vi "add_log_entry.vi"(5 "new entry":string, 6 "error in (no error)":errorcluster, 8 "log identifiers":string(combo), 9 "StatusLog in":refnum<class "StatusLog.lvclass">) -> (0 "error out":errorcluster, 3 "StatusLog out":refnum<class "StatusLog.lvclass">)   [LabVIEW 2017, in "StatusLog.lvclass"]
doc: "adds a new log entry to the logfile. The path to the logfile is internally determined"
uses:
  StatusLog.lvclass
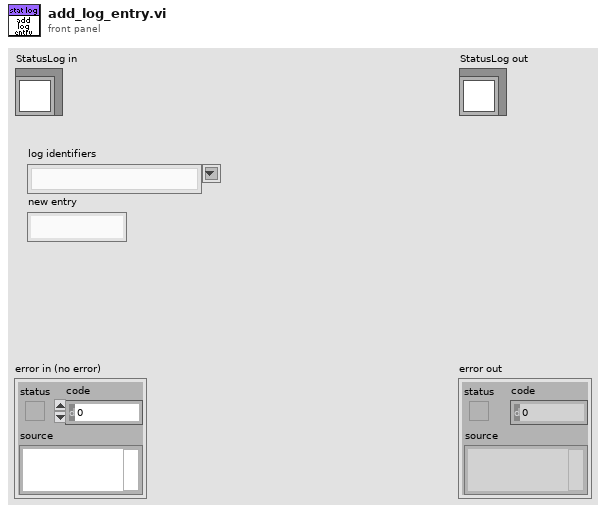
[diagram p1: front panel]
types:
  T1 = enum16{"open", "replace", "create", "open or create", "replace or create", "replace or create with confirmation"}
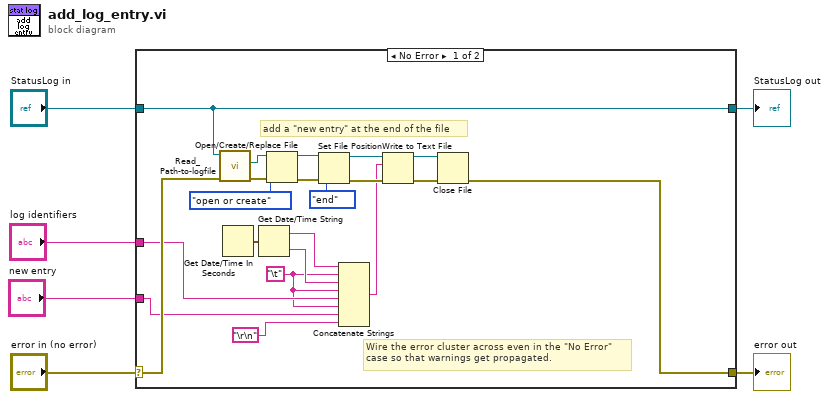
[diagram p0: block diagram]
diagram:
  n1 = case shown="No Error" "error in (no error)" {
    selector: "error in (no error)" -> [w17 w29]
    tunnel: [w16 w29] -> w5
    tunnel: [w27 w28] -> w3
    tunnel: "StatusLog in" -> [w27 w28]
    tunnel: "new entry" -> [w8 _]
    tunnel: "log identifiers" -> [w10 _]
    frame No Error {
      w9 = "\t"
      # "add a \"new entry\" at the end of the file"
      # "Wire the error cluster across even in the \"No Error\"\ncase so that warnings get propagated."
      n2 = call-dynamic "Read_Path-to-logfile.vi"("error in (no error)"=w17, "StatusLog in"=w27) -> ("error out"=w26:errorcluster, "Path to logfile"=w25:path)  [unwired: 7 in, 1 out]
      n3 = Get Date/Time In Seconds() -> (seconds since 1Jan1904=w13:timestamp)
      n4 = Get Date/Time String(seconds (now)=w13) -> (date string=w12:string, time string=w11:string)  [unwired: 2 in]
      n5 = Open/Create/Replace File(file path (use dialog)=w25, error in=w26, operation (0:open)=T1."open or create") -> (refnum out=w23:refnum<file>, error out=w22:errorcluster)  [unwired: 3 in, 1 out]
      n6 = Set File Position(refnum=w23, from (0:start)=enum16{"start", "end", "current"}."end", error in=w22) -> (refnum out=w20:refnum<file>, error out=w24:errorcluster)  [unwired: 1 in]
      n7 = Concatenate Strings(w12, w9, w11, w9, w10, w9, w8, "\r\n") -> (w14:string)
      n8 = Write to Text File(file (use dialog)=w20, text=w14, error in=w24) -> (refnum out=w18:refnum<file>, error out=w19:errorcluster)  [unwired: 1 in, 1 out]
      n9 = Close File(refnum=w18, error in=w19) -> (error out=w16:errorcluster)  [unwired: 1 out]
    }
    frame Error {
    }
  }
  "error out" <- w5
  "StatusLog out" <- w3
